vi "Axis Object Event.vi"(4 "Plot Action":enum16{"Update", "Remove", "Nothing"}(ring), 6 "Axis Action":enum16{"Update", "Remove", "Nothing"}(ring), 8 "error in (no error)":errorcluster, 9 "Object Cluster In":T3, 10 "Actual Transform In":T1, 11 "3D Plot.lvclass in":refnum<class "3D Plot.lvclass">) -> (0 "error out":errorcluster, 1 "Object Cluster Out":T3, 2 "Actual Transform Out":T1, 3 "3D Plot.lvclass out":refnum<class "3D Plot.lvclass">)   [LabVIEW 2020, in "3D Plot.lvclass"]
uses:
  3D Plot.lvclass
  Object Cluster.ctl
  Actual Transform.ctl
  Range Clusters.ctl
  NI_3D Picture Control.lvlib
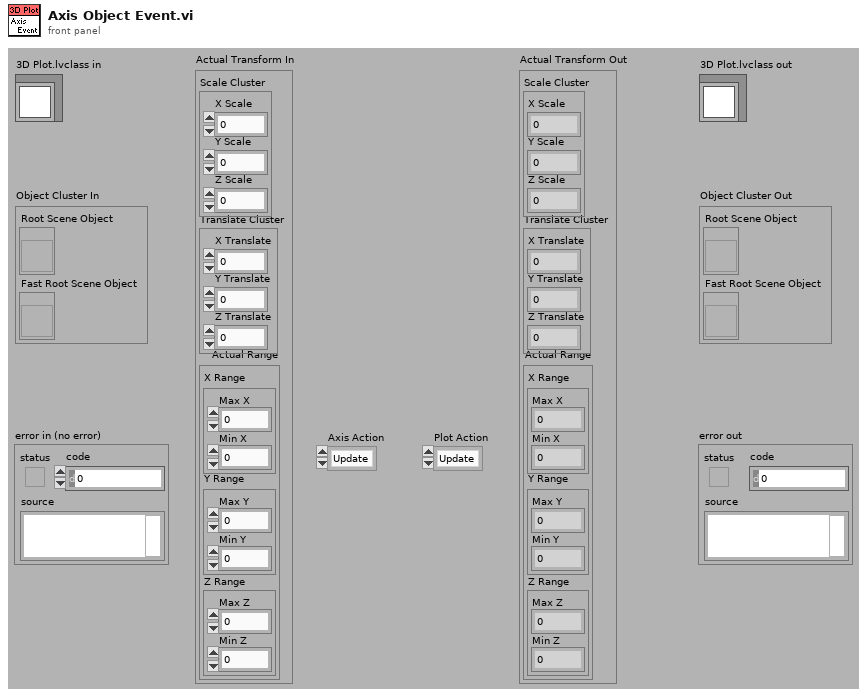
[diagram p1: front panel]
types:
  T1 = typedef "3D Plot.lvclass/Actual Transform.ctl" = cluster{"Scale Cluster":cluster{"X Scale":sgl, "Y Scale":sgl, "Z Scale":sgl}, "Translate Cluster":cluster{"X Translate":sgl, "Y Translate":sgl, "Z Translate":sgl}, "Actual Range":T2}
  T2 = typedef "3D Plot.lvclass/Range Clusters.ctl" = cluster{"X Range":cluster{"Max X":sgl, "Min X":sgl}, "Y Range":cluster{"Max Y":sgl, "Min Y":sgl}, "Z Range":cluster{"Max Z":sgl, "Min Z":sgl}}
  T3 = typedef "3D Plot.lvclass/Object Cluster.ctl" = cluster{"Root Scene Object":refnum<vi>, "Fast Root Scene Object":refnum<vi>}
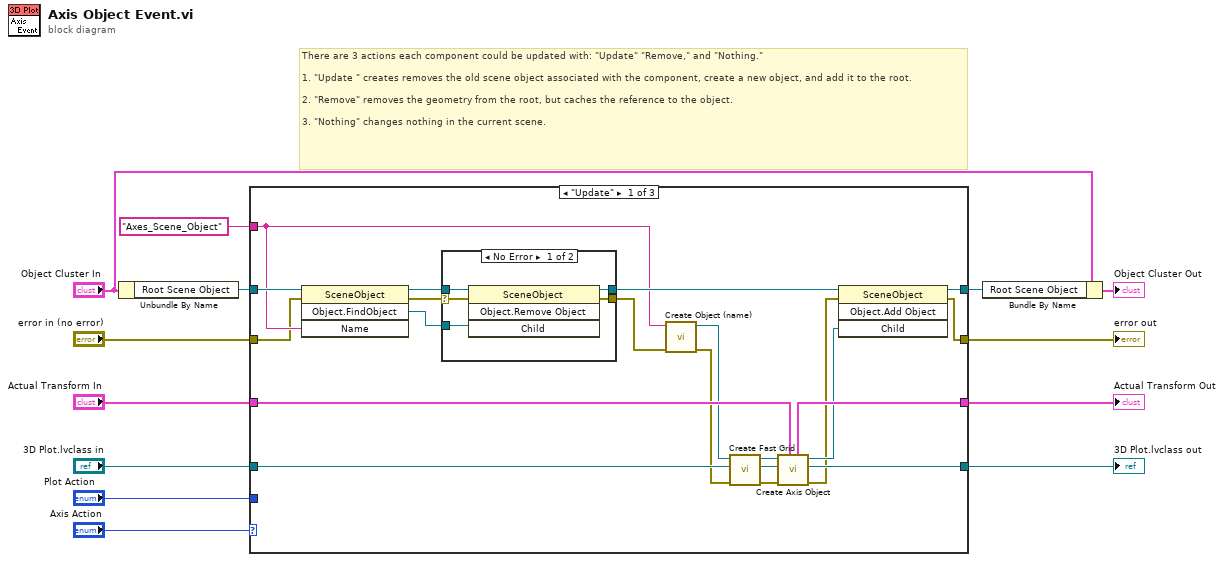
[diagram p0: block diagram]
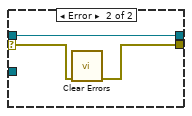
[diagram p2: hidden frame]
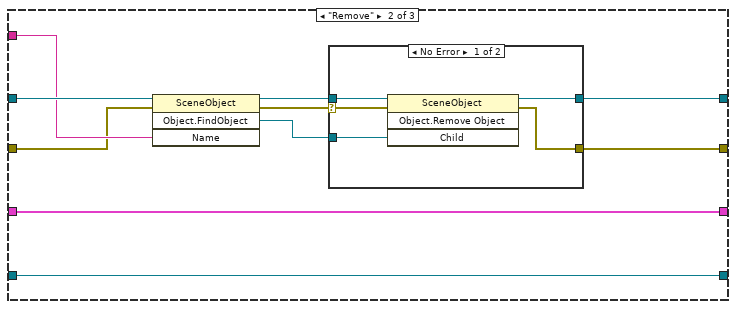
[diagram p3: hidden frame]
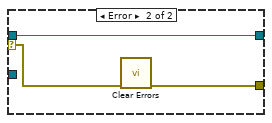
[diagram p4: hidden frame]
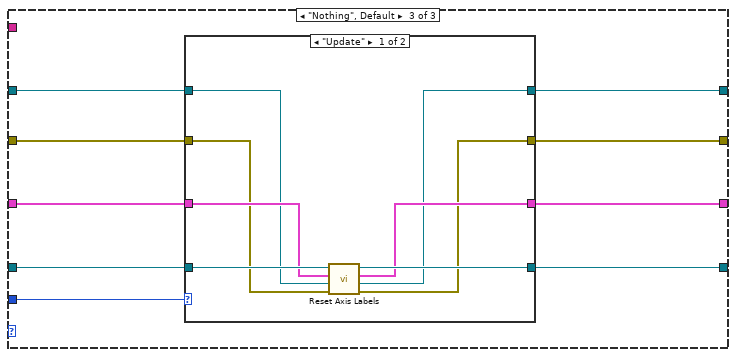
[diagram p5: hidden frame]
diagram:
  # "There are 3 actions each component could be updated with: \"Update\" \"Remove,\" and \"Nothing.\"  \n\n1. \"Update \" creates removes the old scene object associated with the component, create a new object, and add it to the root.  \n\n2. \"Remove\" removes the geometry from the root, but caches the reference to the object.\n\n3. \"Nothing\" changes nothing in the current scene."
  n1 = Unbundle By Name("Object Cluster In") -> ("Root Scene Object"=w6:refnum<vi>)
  n2 = case shown="\"Update\"" "Axis Action" {
    tunnel: "error in (no error)" -> [w15 w44 w65]
    tunnel: [w19 w52 w64] -> w12
    tunnel: [w28 w51 w68] -> w11
    tunnel: "3D Plot.lvclass in" -> [w29 w51 w69]
    tunnel: "Actual Transform In" -> [w27 w50 w67]
    tunnel: [w26 w50 w66] -> w8
    tunnel: w6 -> [w25 w48 w63]
    tunnel: [w20 w49 w62] -> w3
    tunnel: "Axes_Scene_Object" ("Name") -> [w18 w45 _]
    tunnel: "Plot Action" -> [_ _ w61]
    frame "Update" {
      n3 = invoke class="SceneObject" method="Object.FindObject"(reference=w25, error in=w15, "Name"=w18) -> (reference out=w24:refnum<vi>, error out=w14:errorcluster, "FindObject"=w23:refnum<vi>)  [unwired: 1 in, 1 out]
      n4 = case shown="No Error" w14 {
        selector: w14 -> [w35 w41]
        tunnel: [w37 w40] -> w34
        tunnel: w24 -> [w39 w42]
        tunnel: w23 -> [w38 _]
        tunnel: [w36 w42] -> w33
        frame No Error {
          n5 = invoke class="SceneObject" method="Object.Remove Object"(reference=w39, error in=w35, "Child"=w38) -> (reference out=w36:refnum<vi>, error out=w37:errorcluster)  [unwired: 1 in, 2 out]
        }
        frame Error {
          n6 = call "Clear Errors.vi"("error in (no error)"=w41) -> ("error out"=w40:errorcluster)  [unwired: 5 in, 1 out]
        }
      }
      n7 = call "Create Object (name).vi"("error in (no error)"=w34, "Name"=w18) -> ("error out"=w17:errorcluster, "Scene:New Object"=w22:refnum<vi>)  [unwired: 8 in]
      n8 = call "Create Fast Grid.vi"("error in (no error)"=w17, "3D Plot.lvclass in"=w29, "Fast Draw Object In"=w22) -> ("error out"=w32:errorcluster, "3D Plot.lvclass out"=w31:refnum<class "3D Plot.lvclass">, "Fast Draw Object Out"=w30:refnum<vi>)  [unwired: 6 out]
      n9 = call "Create Axis Object.vi"("Actual Transform In"=w27, "error in (no error)"=w32, "3D Plot.lvclass in"=w31, "Axis Object In"=w30) -> ("error out"=w16:errorcluster, "3D Plot.lvclass out"=w28:refnum<class "3D Plot.lvclass">, "Axis Object Out"=w21:refnum<vi>, "Actual Transform Out"=w26:T1)  [unwired: 4 out]
      n10 = invoke class="SceneObject" method="Object.Add Object"(reference=w33, error in=w16, "Child"=w21) -> (reference out=w20:refnum<vi>, error out=w19:errorcluster)  [unwired: 1 in, 2 out]
    }
    frame "Remove" {
      n11 = invoke class="SceneObject" method="Object.FindObject"(reference=w48, error in=w44, "Name"=w45) -> (reference out=w47:refnum<vi>, error out=w43:errorcluster, "FindObject"=w46:refnum<vi>)  [unwired: 1 in, 1 out]
      n12 = case shown="No Error" w43 {
        selector: w43 -> [w53 w59]
        tunnel: w46 -> [w57 _]
        tunnel: w47 -> [w56 w60]
        tunnel: [w55 w60] -> w49
        tunnel: [w54 w58] -> w52
        frame No Error {
          n13 = invoke class="SceneObject" method="Object.Remove Object"(reference=w56, error in=w53, "Child"=w57) -> (reference out=w55:refnum<vi>, error out=w54:errorcluster)  [unwired: 1 in, 2 out]
        }
        frame Error {
          n14 = call "Clear Errors.vi"("error in (no error)"=w59) -> ("error out"=w58:errorcluster)  [unwired: 5 in, 1 out]
        }
      }
    }
    frame "Nothing", Default {
      n15 = case shown="\"Update\"" w61 {
        tunnel: w69 -> [w77 w78]
        tunnel: [w76 w78] -> w68
        tunnel: w67 -> [w75 w79]
        tunnel: [w74 w79] -> w66
        tunnel: w65 -> [w73 w80]
        tunnel: [w72 w80] -> w64
        tunnel: w63 -> [w71 w81]
        tunnel: [w70 w81] -> w62
        frame "Update" {
          n16 = call "Reset Axis Labels.vi"("error in (no error)"=w73, "Root Scene Object out"=w71, "Actual Transform In"=w75, "3D Plot.lvclass in"=w77) -> ("error out"=w72:errorcluster, "Root Scene Object out"=w70:refnum<vi>, "Actual Transform Out"=w74:T1, "3D Plot.lvclass out"=w76:refnum<class "3D Plot.lvclass">)  [unwired: 4 in]
        }
        frame "Nothing", Default {
        }
      }
    }
  }
  "error out" <- w12
  "3D Plot.lvclass out" <- w11
  "Actual Transform Out" <- w8
  n17 = Bundle By Name(cluster="Object Cluster In", "Root Scene Object"=w3) -> (→"Object Cluster Out":T3)
